vi "test Abort Sub2.vi"(11 "Test Case In":refnum<class "Tests Event MessengerM.lvclass">) -> (0 "error out":errorcluster, 3 "Test Case Out":refnum<class "Tests Event MessengerM.lvclass">)   [LabVIEW 2020, in "Tests Event MessengerM.lvclass"]
uses:
  Tests Event MessengerM.lvclass
  C:/Program Files/National Instruments/LabVIEW 2020/vi.lib/Astemes/LUnit/Test Case.lvclass
  <vilib>/Astemes/LUnit/Test Case.lvclass/Test Case.ctl
  <vilib>/Astemes/LUnit/Core/LUnit Test Case/Private/Append Pass Result.vi
  <vilib>/Astemes/LUnit/Core/LUnit Test Case/Private/Append Fail Result.vi
  <vilib>/Astemes/LUnit/Core/LUnit Test Case/Private/Run In UI.vi
  <vilib>/Utility/error.llb/Clear Errors.vi
  <extravilib>/ChannelInstances/Event MessengerM-c(str,var)/Instantiate.vi
  <extravilib>/ChannelInstances/Event MessengerM-c(str,var)/))Channel.vi
  Tests Event MessengerM.lvclass/Tests Event MessengerM.ctl
  <vilib>/Astemes/LUnit/Test Case.lvclass
  <extravilib>/ChannelInstances/Event MessengerM-c(str,var).lvlib
panel:
  out "cmd 2":string
  out "cmd":string
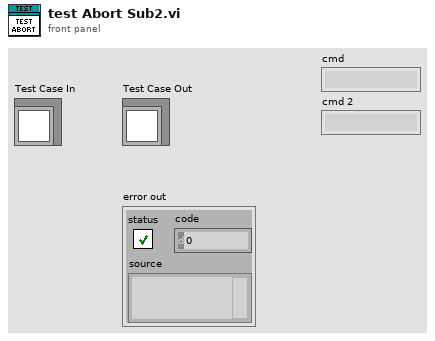
[diagram p1: front panel]
types:
  T1 = typedef "Event MessengerM-c(str,var).lvlib/))Channel.ctl" = refnum<queue>
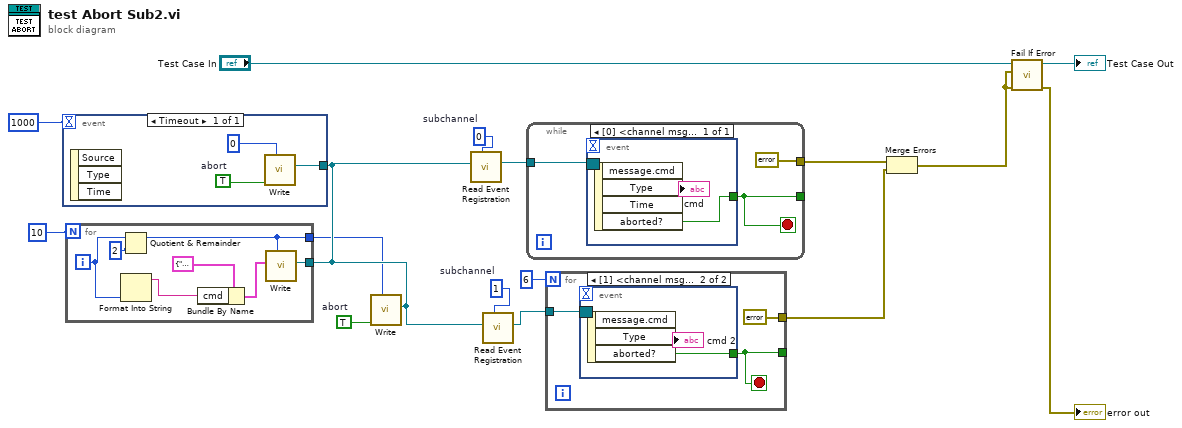
[diagram p0: block diagram]
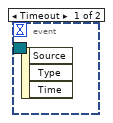
[diagram p2: hidden frame]
diagram:
  w7 = TRUE  # abort
  w3 = 1  # subchannel
  w1 = 0  # subchannel
  n1 = for {
    N: 10 -> [_]
    tunnel: [w18] -> w6
    tunnel: [w17] -> w5
    i -> [w21]
    n2 = Quotient & Remainder(x=w21, y=2) -> (x-y*floor(x/y)=w17:i32)  [unwired: 1 out]
    n3 = Format Into String(w21) -> (resulting string=w20:string)  [unwired: 3 in, 1 out]
    n4 = Bundle By Name(cluster=cluster{"cmd":string, "data":variant} {"cmd"="", "data"=variant} ("element"), "cmd"=w20) -> (w19:cluster{"cmd":string, "data":variant})
    n5 = call <extravilib>:"Write.vi"("subchannel (0)"=w17, "element"=w19) -> ("channel"=w18:T1)  [unwired: 8 in, 1 out]
  }
  n6 = event shown="[0] Timeout" {
    selector: _ -> [_]
    dyn-events: _ -> [_]
    timeout: 1000 -> [_]
    tunnel: w6 -> [w26]
    event Timeout {
      w24 = TRUE  # abort
      n7 = event-data() -> ()  [unwired: 1 in, 3 out]
      n8 = call <extravilib>:"Write.vi"("subchannel (0)"=0, "abort sub (F)"=w24) -> ("channel"=w26:T1)  [unwired: 8 in, 1 out]
    }
  }
  n9 = call <extravilib>:"Write.vi"("channel"=w6, "subchannel (0)"=w5, "abort sub (F)"=w7) -> ()  [unwired: 8 in, 1 out]
  n10 = call <extravilib>:"Read Event Registration.vi"("subchannel (0)"=w1, "channel"=w6) -> ("event registration refnum"=w2:refnum<event-registration>)  [unwired: 9 in]
  n11 = call <extravilib>:"Read Event Registration.vi"("subchannel (0)"=w3, "channel"=w6) -> ("event registration refnum"=w4:refnum<event-registration>)  [unwired: 9 in]
  n12 = while {
    tunnel: w2 -> [w29]
    tunnel: [w28] -> _
    tunnel: [errorcluster {"status"=FALSE, "code"=0, "source"=""} ("error constant")] -> w10
    stop <- w28 stop-if-true
    n13 = event shown="[0] <channel msg>: User Event" {
      selector: w29 -> [_]
      dyn-events: _ -> [_]
      timeout: _ -> [_]
      tunnel: [w30] -> w28
      event User Event {
        n14 = event-data() -> ("message.cmd"=→"cmd":string, "aborted?"=w30:bool)  [unwired: 1 in, 2 out]
      }
    }
  }
  n15 = for {
    N: 6 -> [_]
    tunnel: w4 -> [w34]
    tunnel: [w33] -> _
    tunnel: [errorcluster {"status"=FALSE, "code"=0, "source"=""} ("error constant")] -> w9
    stop <- w33 stop-if-true
    n16 = event shown="[1] <channel msg>: User Event" {
      selector: w34 -> [_ _]
      dyn-events: _ -> [_ _]
      timeout: _ -> [_ _]
      tunnel: [_ w35] -> w33
      event Timeout {
        n17 = event-data() -> ()  [unwired: 1 in, 3 out]
      }
      event User Event {
        n18 = event-data() -> ("message.cmd"=→"cmd 2":string, "aborted?"=w35:bool)  [unwired: 1 in, 1 out]
      }
    }
  }
  n19 = Merge Errors(w10, w9) -> (w8:errorcluster)
  n20 = call <vilib>:"Fail If Error.vi"("error in (no error)"=w8, "Assert error"=w8, "LUnit Test Case In"="Test Case In") -> ("error out"=→"error out":errorcluster, "LUnit Test Case Out"=→"Test Case Out":refnum<class "Tests Event MessengerM.lvclass">)  [unwired: 7 in]
